vi "ENA_Auto Port Extend.vi"(0 "Semiconductor Module Context":T1, 5 "Pins":string[](array[string])=["RF1", "RF2"], 11 "error in (no error)":errorcluster) -> (4 "VISA resource name":refnum<visa-resource-name>, 6 "Semiconductor Module Context Out":T1, 15 "error out":errorcluster)   [LabVIEW 2013]
uses:
  <vilib>/NI_TestStand_SemiconductorModule/NI_TestStand_Semiconductor_Module.lvlibp/PinMap/General/SemiconductorModuleContext.ctl
  Pin Map API/ENA Custom Instrument.lvlib
  <vilib>/NI_TestStand_SemiconductorModule/NI_TestStand_Semiconductor_Module.lvlibp
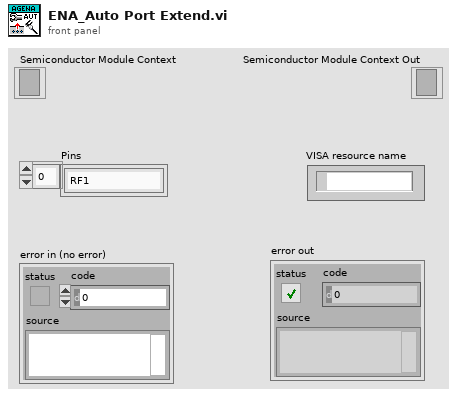
[diagram p1: front panel]
types:
  T1 = typedef "NI_TestStand_Semiconductor_Module.lvlibp/SemiconductorModuleContext.ctl" = refnum<k7>
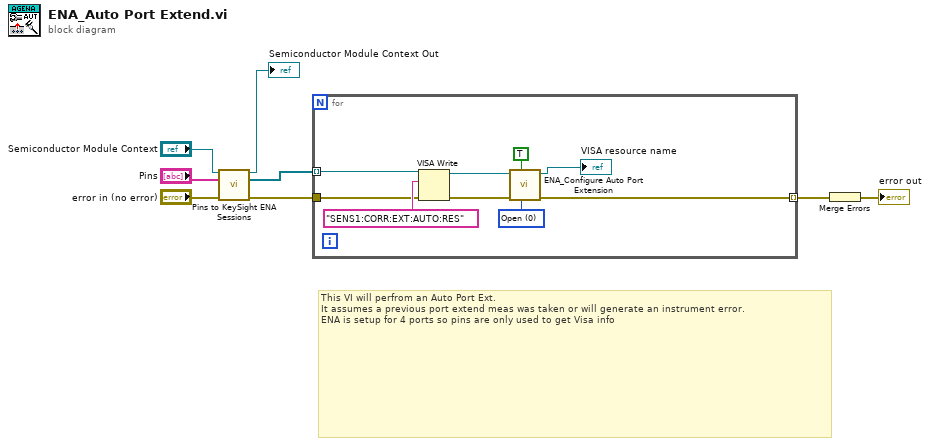
[diagram p0: block diagram]
diagram:
  # "This VI will perfrom an Auto Port Ext.\nIt assumes a previous port extend meas was taken or will generate an instrument error.\nENA is setup for 4 ports so pins are only used to get Visa info"
  n1 = call "Pins to KeySight ENA Sessions.vi"("Semiconductor Module Context"="Semiconductor Module Context", "Pins"="Pins", "error in (no error)"="error in (no error)") -> ("Semiconductor Module Context Out"=→"Semiconductor Module Context Out":T1, "Instrument Sessions"=w6:refnum<visa-resource-name>[], "error out"=w7:errorcluster)  [unwired: 8 in, 2 out]
  n2 = for {
    tunnel: w6 -> [w11] mode=indexing
    tunnel: w7 -> [w12]
    tunnel: [w10] -> w2 mode=indexing
    w14 = 0 items=["Open", "Short"] ("Standard (1: Short)")
    n3 = VISA Write(VISA resource name=w11, write buffer="SENS1:CORR:EXT:AUTO:RES", error in (no error)=w12) -> (VISA resource name out=w15:refnum<visa-resource-name>, error out=w16:errorcluster)  [unwired: 1 out]
    n4 = call "ENA_Configure Auto Port Extension.vi"("Standard (1: Short)"=w14, "Enable Auto Port Extension (T: Enable)"=TRUE, "error in (no error)"=w16, "VISA resource name"=w15) -> ("error out"=w10:errorcluster, "VISA resource name out"=→"VISA resource name":refnum<visa-resource-name>)  [unwired: 6 in]
  }
  n5 = Merge Errors(w2) -> (→"error out":errorcluster)
